vi "Clone Control.vi"(6 "Variant in":variant, 7 "Shift Pressed?":bool, 8 "error in (no error)":errorcluster, 10 "QD Combo Box Ref":refnum<vi>, 11 "QD Launch VI Ref":refnum<vi>) -> (0 "error out":errorcluster, 4 "Variant out":variant)   [LabVIEW 2012, in "Control Operation.lvlib"]
doc: "This Quick Drop Keyboard Shortcut will clone the selected Control(s) or Indicator(s) on the Front Panel but changes Controls to Indicators and vice versa. In addition, if found on the Connector Pane, it will attempt to place the newly created control on the opposite (left / right) side of the Connector Pane.\n\nIt was developed to automate the task where, for example, you have a File Ref (in) control, and you want to wire it through the other side of the ConPane.\n\nNote: This script only supports the following patterns: 4x2x2x4, 5x3x3x5, 6x4x4x6, and 8x6x6x8"
uses:
  Control Operation.lvlib
  <vilib>/regexp/Match Regular Expression.xnode
panel:
  in  "Undo Name":string="Dup Con I/O"
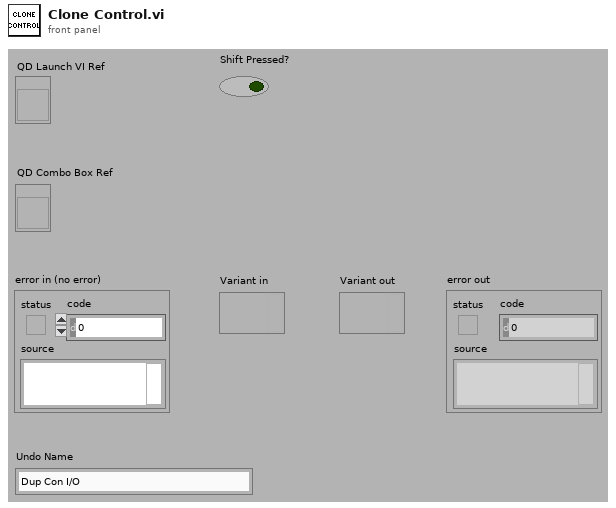
[diagram p1: front panel]
types:
  T1 = typedef "LVPositionTypeDef.ctl" = cluster{"Left":i32, "Top":i32}
  T2 = typedef "LVRectTypeDef.ctl" = cluster{"Left":i16, "Top":i16, "Right":i16, "Bottom":i16}
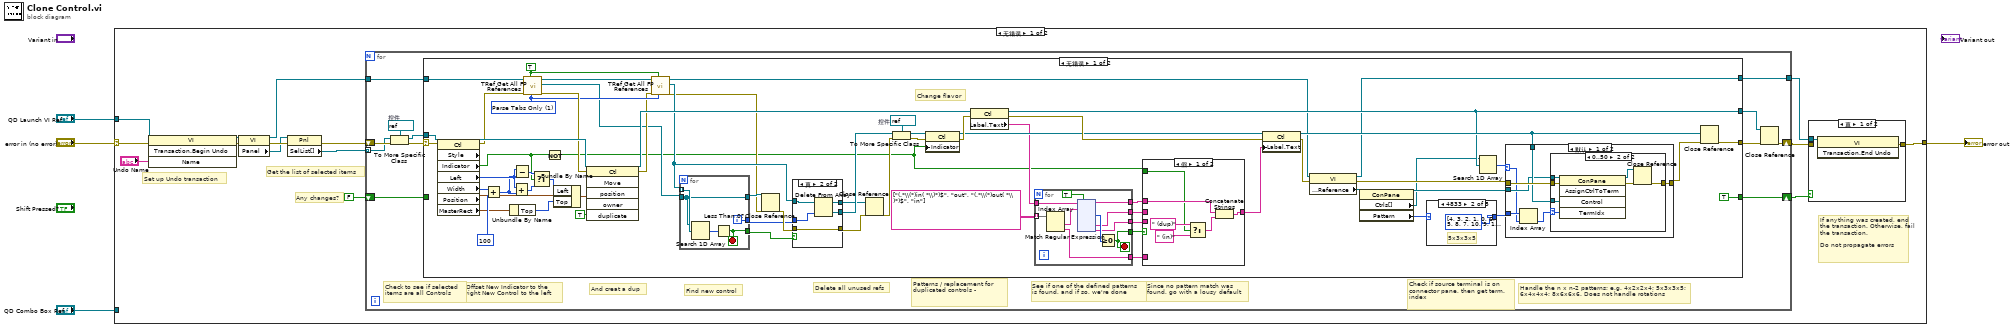
[diagram p0: block diagram]
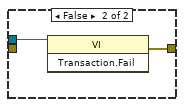
[diagram p2: hidden frame]
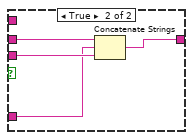
[diagram p3: hidden frame]
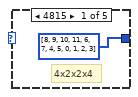
[diagram p5: hidden frame]
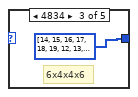
[diagram p6: hidden frame]
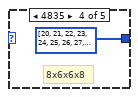
[diagram p7: hidden frame]
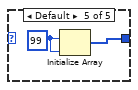
[diagram p8: hidden frame]
diagram:
  n1 = case shown="无错误" "error in (no error)" {
    selector: "error in (no error)" -> [w18 w273]
    tunnel: [w9 w273] -> w1
    tunnel: "QD Combo Box Ref" -> [_ _]
    tunnel: "QD Launch VI Ref" -> [w17 _]
    frame No Error {
      # "If anything was created, end the transaction. Otherwise, fail the transaction.\n\nDo not propagate errors"
      # "Any changes?"
      # "Get the list of selected items"
      # "Set up Undo transaction"
      n2 = invoke class="VI" method="Transaction.Begin Undo"(reference=w17, error in=w18, "Name"="Undo Name") -> (reference out=w5:refnum<vi>, error out=w13:errorcluster)  [unwired: 1 in, 2 out]
      n3 = property class="VI"(reference=w5, error in=w13) -> (reference out=w7:refnum<vi>, error out=w16:errorcluster, "Panel"=w15:refnum<vi>)
      n4 = property class="Pnl"(reference=w15, error in=w16) -> (error out=w8:errorcluster, "SelList[]"=w10:refnum<vi>[])  [unwired: 1 out]
      n5 = for {
        tunnel: w10 -> [w26] mode=indexing
        shift-right: [w28] -> w11
        shift-left: w8 -> [w35]
        shift-right: [w30] -> w12
        shift-left: FALSE -> [w31]
        tunnel: w7 -> [w24]
        tunnel: [w25] -> w6
        w34 = refnum<vi> refnum  # 控件
        # "Since no pattern match was\nfound, go with a lousy default"
        # "Patterns / replacement for duplicated controls -"
        # "Delete all unused refs"
        # "Find new control"
        # "Handle the n x n-2 patterns; e.g. 4x2x2x4; 5x3x3x5;\n6x4x4x4; 8x6x6x6. Does not handle rotations"
        # "Check if source terminal is on\nconnector pane, then get term.\nindex"
        # "See if one of the defined patterns\nis found, and if so, we're done"
        # "And creat a dup"
        # "Offset New Indicator to the\nright New Control to the left"
        # "Check to see if selected\nitems are all Controls"
        n6 = To More Specific Class(target class=w34, reference=w26, error in=w35) -> (specific class reference=w32:refnum<vi>, error out=w33:errorcluster)
        n7 = case shown="无错误" w33 {
          selector: w33 -> [w100 w272]
          tunnel: w32 -> [w73 w271]
          tunnel: [w36 w272] -> w29
          tunnel: [w85 w271] -> w27
          tunnel: [TRUE w270] -> w30
          tunnel: w31 -> [_ w270]
          tunnel: w24 -> [w68 w269]
          tunnel: [w77 w269] -> w25
          frame No Error {
            w59 = refnum<vi> refnum  # 控件
            w62 = u16 1 items=["Parse All", "Parse Tabs Only"] ("Parsing Rule")
            w63 = TRUE ("Ignore Decorations?")
            # "Change flavor"
            n8 = property class="Ctl" props=["Style", "Indicator", "Left", "Width", "Position", "MasterRect"](reference=w73, error in=w100) -> (reference out=w74:refnum<vi>, error out=w67:errorcluster, "Indicator"=w94:bool, "Left"=w96:i32, "Width"=w88:u32, "Position"=w71:T1, "MasterRect"=w70:T2)  [unwired: 1 out]
            n9 = Add(x=w88, y=u32 100 ("x")) -> (x+y=w81:u32)
            n10 = Unbundle By Name(w70) -> ("Top"=w69:i16)
            n11 = Add(x=w96, y=w81) -> (x+y=w97:u32)
            n12 = Subtract(x=w96, y=w81) -> (x-y=w98:u32)
            n13 = call <vilib>:"TRef Get All FP References.vi"("Parsing Rule"=w62, "Ignore Decorations?"=w63, "error in (no error)"=w67, "VI Refnum"=w68) -> ("error out"=w66:errorcluster, "All FP Objects"=w60:refnum<vi>[], "dup VI Refnum"=w65:refnum<vi>)  [unwired: 3 in, 2 out]
            n14 = Select(t=w98, s=w94, f=w97) -> (s? t:f=w95:u32)
            n15 = Not(x=w94) -> (.not. x?=w40:bool)
            n16 = Bundle By Name(cluster=w71, "Left"=w95, "Top"=w69) -> (w76:T1)
            n17 = invoke class="Ctl" method="Move"(reference=w74, error in=w66, "position"=w76, "duplicate"=TRUE ("Duplicate? (F)")) -> (reference out=w72:refnum<vi>, error out=w61:errorcluster)  [unwired: 2 in, 4 out]
            n18 = call <vilib>:"TRef Get All FP References.vi"("Parsing Rule"=w62, "Ignore Decorations?"=w63, "error in (no error)"=w61, "VI Refnum"=w65) -> ("error out"=w47:errorcluster, "All FP Objects"=w54:refnum<vi>[], "dup VI Refnum"=w64:refnum<vi>)  [unwired: 3 in, 2 out]
            n19 = for {
              tunnel: w60 -> [w243]
              tunnel: w54 -> [w244] mode=indexing
              tunnel: [w245] -> w55
              tunnel: [w243] -> w57
              tunnel: [w242] -> w53
              i -> [w242]
              stop <- w245 stop-if-true
              n20 = Search 1D Array(1D array=w243, element=w244) -> (index of element=w246:i32)  [unwired: 1 in]
              n21 = Less Than 0?(x=w246) -> (x < 0?=w245:bool)
            }
            n22 = Close Reference(reference=w57, error in (no error)=w47) -> (error out=w56:errorcluster)
            n23 = case shown="真" w55 {
              tunnel: w56 -> [w235 w237]
              tunnel: w54 -> [w236 w241]
              tunnel: w53 -> [_ w240]
              tunnel: [_ w239] -> w52
              tunnel: [w236 w238] -> w51
              tunnel: [w235 w237] -> w50
              frame False {
              }
              frame True {
                n24 = Delete From Array(array=w241, index=w240) -> (deleted portion=w239:refnum<vi>, array with subset deleted=w238:refnum<vi>[])  [unwired: 1 in]
              }
            }
            n25 = Close Reference(reference=w51, error in (no error)=w50) -> (error out=w49:errorcluster)
            n26 = To More Specific Class(target class=w59, reference=w52, error in=w49) -> (specific class reference=w58:refnum<vi>, error out=w48:errorcluster)
            n27 = property class="Ctl"(reference=w58, error in=w48, "Indicator"=w40) -> (reference out=w91:refnum<vi>, error out=w92:errorcluster)
            n28 = property class="Ctl"(reference=w72, error in=w92) -> (reference out=w85:refnum<vi>, error out=w93:errorcluster, "Label.Text"=w45:string)
            n29 = for {
              tunnel: w45 -> [w118]
              tunnel: string[][] [["(.*\\(*)in( *\\)*)$", "out"], ["(.*\\(*)out( *\\)*)$", "in"]] ("Match") -> [w120] mode=indexing
              tunnel: [w119] -> w43
              tunnel: [w115] -> w42
              tunnel: [w114] -> w39
              tunnel: [w113] -> w38
              tunnel: [w112] -> w37
              stop <- w119 stop-if-true
              n30 = Index Array(array=w120) -> (element #1=w117:string, element #2=w114:string)  [unwired: 2 in]
              n31 = xnode "Match Regular Expression"("输入字符串"=w118, "正则表达式"=w117, "忽略大小写？(F)"=TRUE ("ignore case? (F)")) -> ("匹配之前"=w115:string, "匹配后偏移量"=w116:i32, "子匹配 1"=w113:string, "子匹配 2"=w112:string)  [unwired: 3 in, 3 out]
              n32 = Greater Or Equal To 0?(x=w116) -> (x >= 0?=w119:bool)
            }
            n33 = case shown="假" w43 {
              tunnel: w42 -> [w103 _]
              tunnel: [w102 w110] -> w41
              tunnel: w40 -> [w101 _]
              tunnel: w39 -> [_ w107]
              tunnel: w38 -> [_ w109]
              tunnel: w37 -> [_ w108]
              frame False {
                n34 = Select(t=" (dup)" ("string"), s=w101, f=" (in)" ("string")) -> (s? t:f=w106:string)
                n35 = Concatenate Strings(w103, w106) -> (w102:string)
              }
              frame True {
                n36 = Concatenate Strings(w109, w107, w108) -> (w110:string)
              }
            }
            n37 = property class="Ctl"(reference=w91, error in=w93, "Label.Text"=w41) -> (reference out=w89:refnum<vi>, error out=w83:errorcluster)
            n38 = property class="VI"(reference=w64, error in=w83) -> (reference out=w77:refnum<vi>, error out=w90:errorcluster, "Connector Pane:Reference"=w87:refnum<vi>)
            n39 = property class="ConPane"(reference=w87) -> (reference out=w86:refnum<vi>, "Ctrls[]"=w46:refnum<vi>[], "Pattern"=w79:u32)  [unwired: 1 in, 1 out]
            n40 = case shown="4833" w79 {
              tunnel: [u32[] [8, 9, 10, 11, 6, 7, 4, 5, 0, 1, 2, 3] u32[] [4, 3, 2, 1, 0, 6, 5, 8, 7, 10, 9, 15, 14, 13, 12, 11] u32[] [14, 15, 16, 17, 18, 19, 12, 13, 10, 11, 8, 9, 6, 7, 0, 1, 2, 3, 4, 5] u32[] [20, 21, 22, 23, 24, 25, 26, 27, 18, 19, 16, 17, 14, 15, 12, 13, 10, 11, 8, 9, 0, 1, 2, 3, 4, 5, 6, 7] w252] -> w78
              frame 4815 {
                # "4x2x2x4"
              }
              frame 4833 {
                # "5x3x3x5"
              }
              frame 4834 {
                # "6x4x4x6"
              }
              frame 4835 {
                # "8x6x6x8"
              }
              frame Default {
                w251 = u32 99 ("Terminal Index")
                n41 = Initialize Array(w251, w251) -> (w252:u32[])
              }
            }
            n42 = Search 1D Array(1D array=w46, element=w85) -> (index of element=w84:i32)  [unwired: 1 in]
            n43 = case shown="默认" w84 {
              selector: w84 -> [w254 _]
              tunnel: w90 -> [w259 w268]
              tunnel: w89 -> [w258 _]
              tunnel: w86 -> [w257 _]
              tunnel: [w256 w268] -> w82
              tunnel: w78 -> [w255 _]
              frame Default {
                n44 = Index Array(array=w255, index=w254) -> (element=w253:u32)
                n45 = case shown="0..50" w253 {
                  selector: w253 -> [_ w263]
                  tunnel: w259 -> [w260 w267]
                  tunnel: w258 -> [_ w266]
                  tunnel: w257 -> [_ w265]
                  tunnel: [w260 w262] -> w256
                  frame 99, Default {
                  }
                  frame 0..50 {
                    n46 = invoke class="ConPane" method="AssignCtrlToTerm"(reference=w265, error in=w267, "Control"=w266, "TermIdx"=w263) -> (reference out=w261:refnum<vi>, error out=w264:errorcluster)  [unwired: 1 in, 3 out]
                    n47 = Close Reference(reference=w261, error in (no error)=w264) -> (error out=w262:errorcluster)
                  }
                }
              }
              frame -1 {
              }
            }
            n48 = Close Reference(reference=w89, error in (no error)=w82) -> (error out=w36:errorcluster)
          }
          frame Error {
          }
        }
        n49 = Close Reference(reference=w27, error in (no error)=w29) -> (error out=w28:errorcluster)
      }
      n50 = case shown="真" w12 {
        tunnel: w11 -> [_ _]
        tunnel: w6 -> [w20 w22]
        tunnel: [w21 w23] -> w9
        frame True {
          n51 = invoke class="VI" method="Transaction.End Undo"(reference=w20) -> (error out=w21:errorcluster)  [unwired: 2 in, 2 out]
        }
        frame False {
          n52 = invoke class="VI" method="Transaction.Fail"(reference=w22) -> (error out=w23:errorcluster)  [unwired: 2 in, 2 out]
        }
      }
    }
    frame Error {
    }
  }
  "error out" <- w1
